vi "Class Operator-Traverse.vi"(7 "Traverse All":bool, 8 "error in (no error)":errorcluster, 9 "Context Data":variant, 10 "Operator Name":string, 11 "Generic in":refnum<class "Generic.lvclass">) -> (0 "error out":errorcluster, 1 "Context Data 2":variant, 2 "Class Operator:Traverse":bool, 3 "Generic out":refnum<class "Generic.lvclass">)   [LabVIEW 2020, in "Generic.lvclass"]
doc: "Traverses the object tree of a specified object and performs a function on any object that has a process specified. If the traverse fails, LabVIEW returns FALSE.\n\n Traverse is a way to find object references without having to recursively find them in a VI or block diagram.\n\n\n<b>Caution</b> Do not attempt to modify code in traverse callbacks. This changes the stack the traverse operation is iterating through and can cause LabVIEW to crash.\n\nQControl Class wrapper around the <b>Generic : Class Operator:Traverse Method</b>.\n<b> </b> <b> </b>\n©2016 Q Software Innovations, LLC (QSI)\nwritten by Quentin Alldredge\nproduced in LabVIEW 2015\n\nsupport@qsoftwareinnovations.com\nwww.qsoftwareinnovations.com\n\nAll rights reserved.\n\nRedistribution and use in source and binary forms, with or without modification, are permitted provided that the following conditions are met:\n\n * Redistributions of source code must retain the above copyright notice, this list of conditions and the following disclaimer.\n * Redistributions in binary form must reproduce the above copyright notice, this list of conditions and the following disclaimer in the documentation and/or other materials provided with the distribution.\n * Neither the name of Q Software Innovations, LLC. nor the names of its contributors may be used to endorse or promote products derived from this software without specific prior written permission.\n\nTHIS SOFTWARE IS PROVIDED BY THE COPYRIGHT HOLDERS AND CONTRIBUTORS \"AS IS\" AND ANY EXPRESS OR IMPLIED WARRANTIES, INCLUDING, BUT NOT LIMITED TO, THE IMPLIED WARRANTIES OF MERCHANTABILITY AND FITNESS FOR A PARTICULAR PURPOSE ARE DISCLAIMED. IN NO EVENT SHALL THE COPYRIGHT OWNER OR CONTRIBUTORS BE LIABLE FOR ANY DIRECT, INDIRECT, INCIDENTAL, SPECIAL, EXEMPLARY, OR CONSEQUENTIAL DAMAGES (INCLUDING, BUT NOT LIMITED TO, PROCUREMENT OF SUBSTITUTE GOODS OR SERVICES; LOSS OF USE, DATA, OR PROFITS; OR BUSINESS INTERRUPTION) HOWEVER CAUSED AND ON ANY THEORY OF LIABILITY, WHETHER IN CONTRACT, STRICT LIABILITY, OR TORT (INCLUDING NEGLIGENCE OR OTHERWISE) ARISING IN ANY WAY OUT OF THE USE OF THIS SOFTWARE, EVEN IF ADVISED OF THE POSSIBILITY OF SUCH DAMAGE."
uses:
  Generic.lvclass
  Generic.lvclass/Generic.ctl
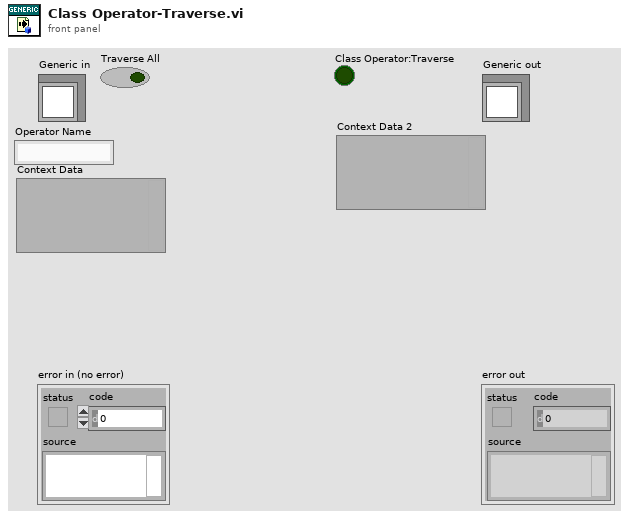
[diagram p1: front panel]
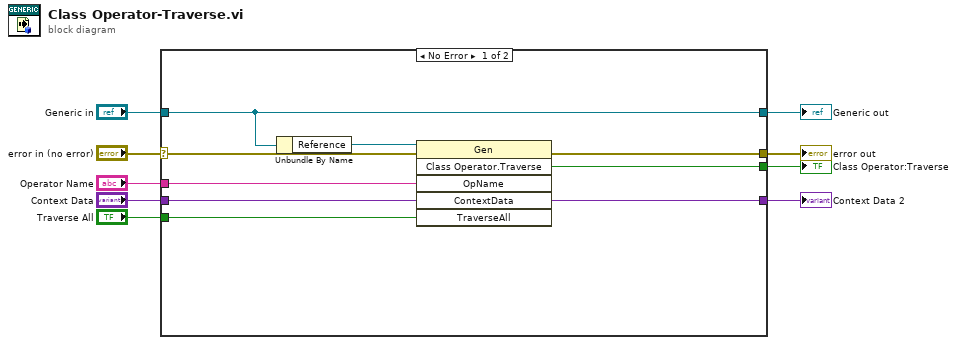
[diagram p0: block diagram]
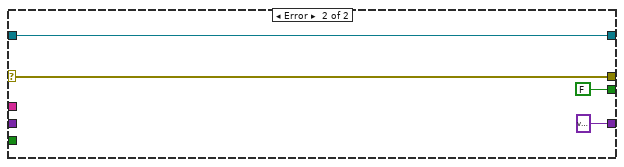
[diagram p2: hidden frame]
diagram:
  n1 = case shown="No Error" "error in (no error)" {
    selector: "error in (no error)" -> [w18 w22]
    tunnel: [w17 w22] -> w8
    tunnel: [w16 w21] -> w6
    tunnel: "Generic in" -> [w16 w21]
    tunnel: "Operator Name" -> [w14 _]
    tunnel: [w13 FALSE ("Traverse")] -> w4
    tunnel: "Context Data" -> [w12 _]
    tunnel: [w11 variant ("ContextData")] -> w2
    tunnel: "Traverse All" -> [w10 _]
    frame No Error {
      n2 = Unbundle By Name(w16) -> ("Reference"=w15:refnum<vi>)
      n3 = invoke class="Gen" method="Class Operator.Traverse"(reference=w15, error in=w18, "OpName"=w14, "ContextData"=w12, "TraverseAll"=w10) -> (error out=w17:errorcluster, "Traverse"=w13:bool, "ContextData"=w11:variant)  [unwired: 1 in, 3 out]
    }
    frame Error {
    }
  }
  "error out" <- w8
  "Generic out" <- w6
  "Class Operator:Traverse" <- w4
  "Context Data 2" <- w2
